vi "Vision Research Phantom Series Initialize.vi"(1 "Storage Path (\"\")":path=path "C:/ProgramData/Phantom/788", 5 "error in (no error)":errorcluster, 7 "CallID":u32, 9 "ID Query (T: Check)":bool, 11 "Reset (F: Don't Reset)":bool) -> (15 "Returned String":string, 19 "Error Out":errorcluster)   [LabVIEW 2013, in "VRI.lvlib"]
doc: "This VI is used to establish communication with a Vision Research Phantom Series camera. The function has an instrument descriptor string as an input. Also, the VI can perform user selectable ID query and/or reset operations.\n\nYou must run this VI before using any of the data, utility, or application example VIs for this device.\n\nWritten by:\nBLOOMY CONTROLS, INC\nWINDSOR, CT 06095, USA\n860-298-9925\nwww.bloomy.com\nV1.0.0\nMay, 2004"
uses:
  VRI.lvlib
panel:
  # "For instructions on the use of this VI, press Ctrl+H to display the help window and move the mouse over the icon, controls, and indicators"
  # "Check\n\n\nDon't Check"
  # "Reset \n\nDon't Reset"
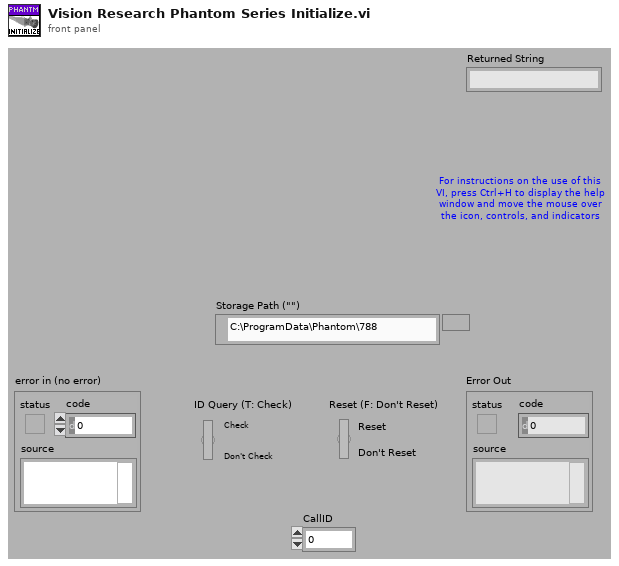
[diagram p1: front panel]
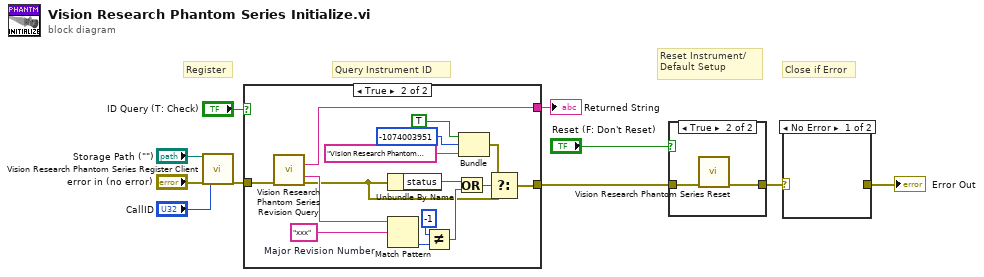
[diagram p0: block diagram]
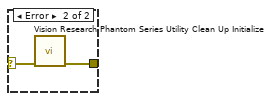
[diagram p2: hidden frame]
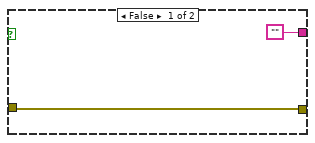
[diagram p4: hidden frame]
diagram:
  # "Close if Error"
  # "Query Instrument ID"
  # "Reset Instrument/\nDefault Setup"
  # "Register"
  n1 = call "Vision Research Phantom Series Register Client.vi"("Storage Path (\"\")"="Storage Path (\"\")", "Error In (no error)"="error in (no error)", "CallID"="CallID") -> ("Error Out"=w3:errorcluster)  [unwired: 16 out]
  n2 = case shown="True" "ID Query (T: Check)" {
    tunnel: [w12 w27] -> w10
    tunnel: w3 -> [w12 w18]
    tunnel: ["" w15] -> w6
    frame False {
    }
    frame True {
      w16 = "xxx"  # Major Revision Number
      n3 = call "Vision Research Phantom Series Revision Query.vi"("Error In (no error)"=w18) -> ("Returned String"=w15:string, "Instr Firmware Revision"=w17:string, "Error Out"=w14:errorcluster)  [unwired: 12 out]
      n4 = Unbundle By Name(w14) -> ("status"=w23:bool)
      n5 = Match Pattern(string=w17, regular expression=w16) -> (offset past match=w21:i32)  [unwired: 4 out]
      n6 = Not Equal?(x=-1, y=w21) -> (x != y?=w25:bool)
      n7 = Or(x=w23, y=w25) -> (x .or. y?=w24:bool)
      n8 = Bundle(TRUE, -1074003951, "VI Name"="Vision Research Phantom Series Initialize") -> (w13:cluster{bool, i32, "VI Name":string})  [unwired: 1 out]
      n9 = Select(t=w13, s=w24, f=w14) -> (s? t:f=w27:errorcluster)
    }
  }
  "Returned String" <- w6
  n10 = case shown="True" "Reset (F: Don't Reset)" {
    tunnel: w10 -> [w28 w29]
    tunnel: [w28 w30] -> w5
    frame False {
    }
    frame True {
      n11 = call "Vision Research Phantom Series Reset.vi"("Error In (no error)"=w29) -> ("Error Out"=w30:errorcluster)  [unwired: 1 in, 13 out]
    }
  }
  n12 = case shown="No Error" w5 {
    selector: w5 -> [_ w31]
    tunnel: [_ w32] -> w7
    frame No Error {
    }
    frame Error {
      n13 = call "Vision Research Phantom Series Utility Clean Up Initialize.vi"("Error In (no error)"=w31) -> ("Error Out"=w32:errorcluster)  [unwired: 1 in, 13 out]
    }
  }
  "Error Out" <- w7
